vi "DAC9767模块换算.vi"(1 "电压精度":u8, 2 "最低电压":dbl, 3 "最高电压":dbl, 4 "数值":dbl) -> (0 "换算16进制":u16)   [LabVIEW 2017]
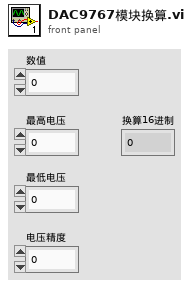
[diagram p1: front panel]
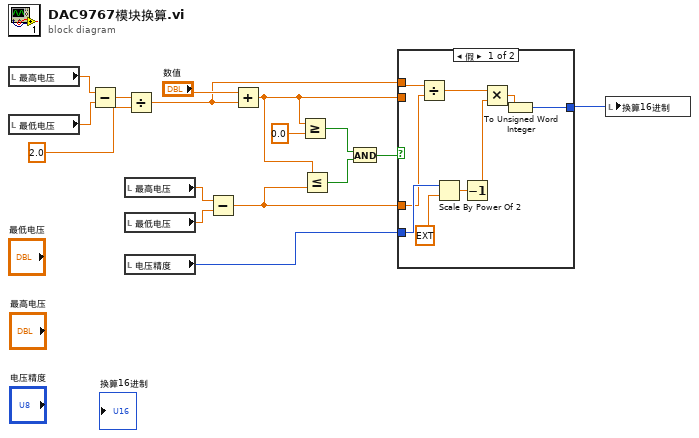
[diagram p0: block diagram]
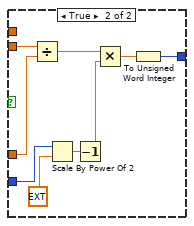
[diagram p2: hidden frame]
diagram:
  n1 = local read "最高电压"() -> (w10:dbl)
  n2 = local read "最低电压"() -> (w9:dbl)
  n3 = Subtract(x=w10, y=w9) -> (x-y=w8:dbl)
  n4 = local read "最高电压"() -> (w6:dbl)
  n5 = local read "最低电压"() -> (w5:dbl)
  n6 = local read "电压精度"() -> (w3:u8)
  n7 = Divide(x=w8, y=2.0) -> (x/y=w1:dbl)
  n8 = Subtract(x=w6, y=w5) -> (x-y=w4:dbl)
  n9 = Add(x="数值", y=w1) -> (x+y=w11:dbl)
  n10 = Greater Or Equal?(x=w11, y=0.0) -> (x >= y?=w14:bool)
  n11 = Less Or Equal?(x=w11, y=w4) -> (x <= y?=w13:bool)
  n12 = And(x=w14, y=w13) -> (x .and. y?=w12:bool)
  n13 = case shown="假" w12 {
    tunnel: w11 -> [_ w34]
    tunnel: w4 -> [w20 w33]
    tunnel: w3 -> [w22 w31]
    tunnel: [w25 w28] -> w2
    tunnel: w1 -> [w21 _]
    frame False {
      n14 = Divide(x=w21, y=w20) -> (x/y=w24:dbl)
      n15 = Scale By Power Of 2(n=w22, x=ext 1.0) -> (x*2^n=w18:ext)
      n16 = Decrement(x=w18) -> (x-1=w17:ext)
      n17 = Multiply(x=w24, y=w17) -> (x*y=w19:ext)
      n18 = To Unsigned Word Integer(number=w19) -> (unsigned 16bit integer=w25:u16)
    }
    frame True {
      n19 = Divide(x=w34, y=w33) -> (x/y=w32:dbl)
      n20 = Scale By Power Of 2(n=w31, x=ext 1.0) -> (x*2^n=w27:ext)
      n21 = Decrement(x=w27) -> (x-1=w26:ext)
      n22 = Multiply(x=w32, y=w26) -> (x*y=w29:ext)
      n23 = To Unsigned Word Integer(number=w29) -> (unsigned 16bit integer=w28:u16)
    }
  }
  n24 = local write "换算16进制"(w2) -> ()
